vi "Read All.vi"(8 "error in":errorcluster, 11 "VISA resource name":refnum<visa-resource-name>) -> (0 "error out":errorcluster, 2 "Message":string, 3 "VISA resource name out":refnum<visa-resource-name>)   [LabVIEW 2019, in "Andeen-Hagerling 2700(400 firmware).lvlib"]
doc: "Read all characters until from the selected VISA resource until no more are available."
uses:
  Andeen-Hagerling 2700(400 firmware).lvlib
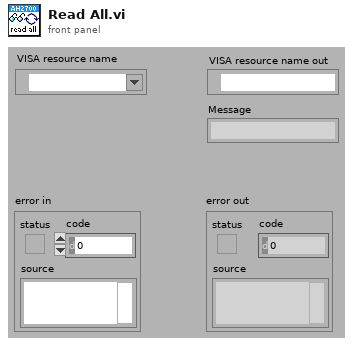
[diagram p1: front panel]
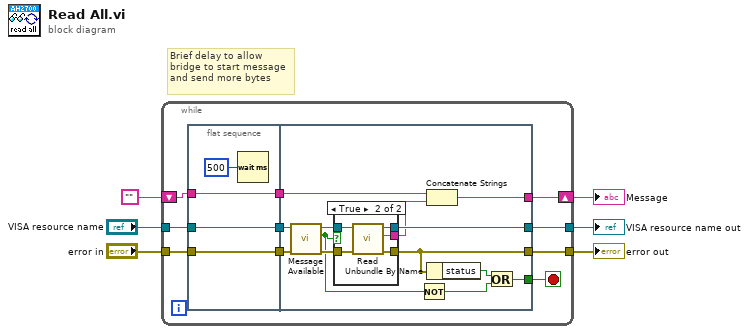
[diagram p0: block diagram]
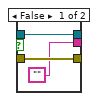
[diagram p2: hidden frame]
diagram:
  # "Brief delay to allow\nbridge to start message\nand send more bytes"
  n1 = while {
    tunnel: "error in" -> [w16]
    tunnel: "VISA resource name" -> [w15]
    tunnel: [w13] -> w3
    tunnel: [w14] -> w2
    shift-right: [w11] -> w1
    shift-left: "" -> [w12]
    stop <- w10 stop-if-true
    n2 = flat-sequence {
      tunnel: w12 -> [w18]
      tunnel: w15 -> [w19]
      tunnel: w16 -> [w20]
      tunnel: [w20] -> w9
      tunnel: [w19] -> w8
      tunnel: [w18] -> w7
      tunnel: [w29] -> w14
      tunnel: [w21] -> w13
      tunnel: [w26] -> w11
      tunnel: [w22] -> w10
      tunnel: w9 -> [w33]
      tunnel: w8 -> [w32]
      tunnel: w7 -> [w27]
      frame #0 {
        n3 = Wait (ms)(milliseconds to wait=u32 500) -> ()  [unwired: 1 out]
      }
      frame #1 {
        n4 = call "Message Available.vi"("error in"=w33, "VISA resource name"=w32) -> ("error out"=w30:errorcluster, "message available"=w24:bool, "VISA resource name out"=w31:refnum<visa-resource-name>)  [unwired: 7 in]
        n5 = case shown="True" w24 {
          tunnel: w31 -> [w36 w41]
          tunnel: w30 -> [w35 w40]
          tunnel: ["" w39] -> w28
          tunnel: [w36 w38] -> w29
          tunnel: [w35 w37] -> w21
          frame False {
          }
          frame True {
            n6 = call "Read.vi"("error in"=w40, "VISA resource name"=w41) -> ("error out"=w37:errorcluster, "Message"=w39:string, "VISA resource name out"=w38:refnum<visa-resource-name>)  [unwired: 7 in]
          }
        }
        n7 = Not(x=w24) -> (.not. x?=w23:bool)
        n8 = Concatenate Strings(w27, w28) -> (w26:string)
        n9 = Unbundle By Name(w21) -> ("status"=w25:bool)
        n10 = Or(x=w25, y=w23) -> (x .or. y?=w22:bool)
      }
    }
  }
  "VISA resource name out" <- w2
  "error out" <- w3
  "Message" <- w1
